vi "test-bang-bang-tolerance.vi"(8 "error in (no error)":errorcluster) -> (0 "error out":errorcluster, 3 "All Tests Passed":bool)   [LabVIEW 2019]
uses:
  <vilib>/Rock Robotics/WPI/ThirdParty/JAS_Junk/TrajLib/BangBang_SetTolerance.vi
  <vilib>/Rock Robotics/WPI/ThirdParty/JAS_Junk/TrajLib/Trajectory_Library.lvlib
panel:
  out "Test Passed 1":bool
  out "Test Passed 0":bool
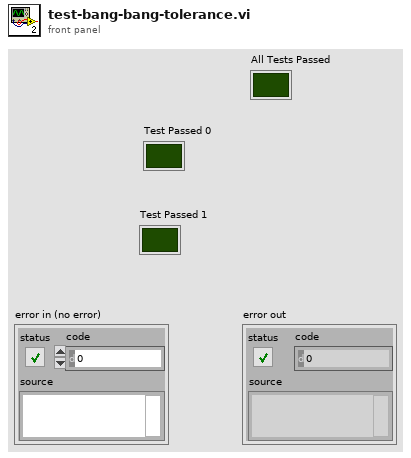
[diagram p1: front panel]
types:
  T1 = typedef "Trajectory_Library.lvlib/BANG_BANG.ctl" = cluster{"Tolerance":dbl, "Setpoint":dbl, "Measurment":dbl}
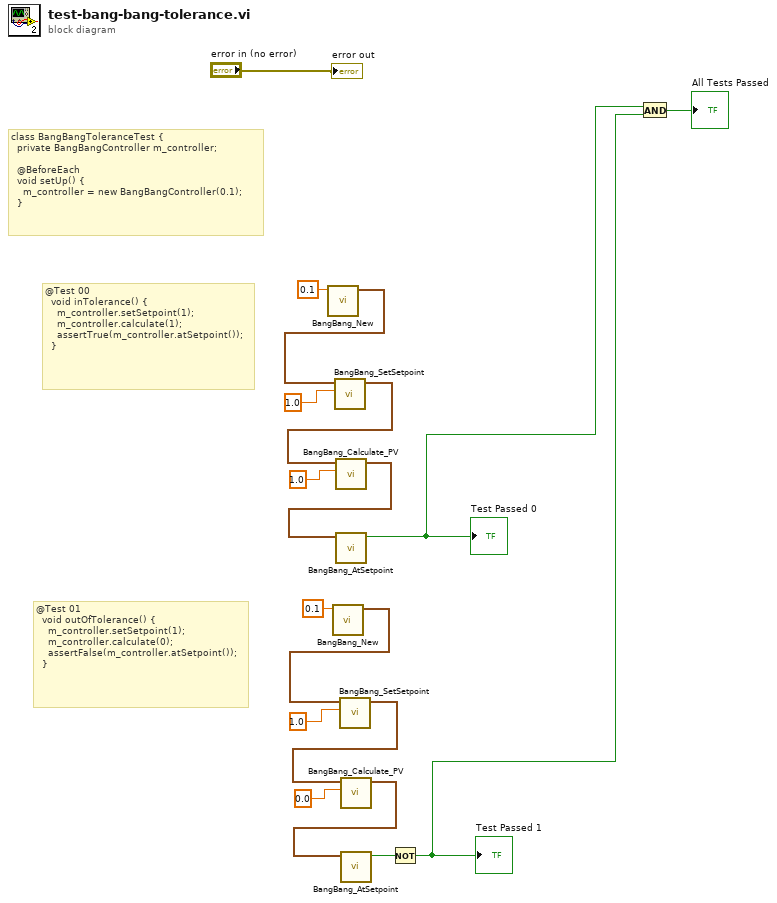
[diagram p0: block diagram]
diagram:
  # "@Test 01\n  void outOfTolerance() {\n    m_controller.setSetpoint(1);\n    m_controller.calculate(0);\n    assertFalse(m_controller.atSetpoint());\n  }"
  # "@Test 00\n  void inTolerance() {\n    m_controller.setSetpoint(1);\n    m_controller.calculate(1);\n    assertTrue(m_controller.atSetpoint());\n  }"
  # "class BangBangToleranceTest {\n  private BangBangController m_controller;\n\n  @BeforeEach\n  void setUp() {\n    m_controller = new BangBangController(0.1);\n  }"
  n1 = call <vilib>:"BangBang_New.vi"("Tolerance"=0.1) -> ("BANG_BANG"=w16:T1)  [unwired: 10 in]
  n2 = call <vilib>:"BangBang_New.vi"("Tolerance"=0.1) -> ("BANG_BANG"=w10:T1)  [unwired: 10 in]
  n3 = call <vilib>:"BangBang_SetSetpoint.vi"("Setpoint"=1.0, "BANG_BANG"=w16) -> ("out BANG_BANG"=w14:T1)  [unwired: 9 in]
  n4 = call <vilib>:"BangBang_Calculate_PV.vi"("Measurment"=1.0, "BANG_BANG"=w14) -> ("out BANG_BANG"=w12:T1)  [unwired: 8 in, 1 out]
  n5 = call <vilib>:"BangBang_AtSetpoint.vi"("BANG_BANG"=w12) -> ("AtSetpoint"=w2:bool)  [unwired: 10 in]
  "Test Passed 0" <- w2
  n6 = call <vilib>:"BangBang_SetSetpoint.vi"("Setpoint"=1.0, "BANG_BANG"=w10) -> ("out BANG_BANG"=w8:T1)  [unwired: 9 in]
  n7 = call <vilib>:"BangBang_Calculate_PV.vi"("Measurment"=0.0, "BANG_BANG"=w8) -> ("out BANG_BANG"=w6:T1)  [unwired: 8 in, 1 out]
  n8 = call <vilib>:"BangBang_AtSetpoint.vi"("BANG_BANG"=w6) -> ("AtSetpoint"=w5:bool)  [unwired: 10 in]
  n9 = Not(x=w5) -> (.not. x?=w1:bool)
  "Test Passed 1" <- w1
  n10 = And(x=w2, y=w1) -> (x .and. y?=→"All Tests Passed":bool)
  "error out" <- "error in (no error)"
